vi "Front Lifter Control.vi"(11 "Go to Level?":i32) -> ()   [LabVIEW 2014]
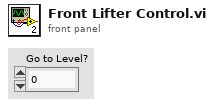
[diagram p1: front panel]
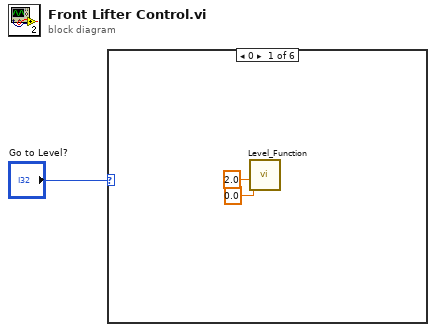
[diagram p0: block diagram]
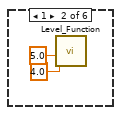
[diagram p2: hidden frame]
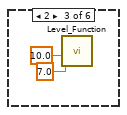
[diagram p3: hidden frame]
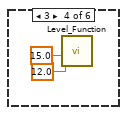
[diagram p4: hidden frame]
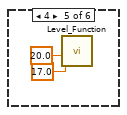
[diagram p5: hidden frame]
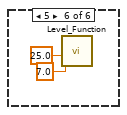
[diagram p6: hidden frame]
diagram:
  n1 = case shown="0" "Go to Level?" {
    frame 0 {
      n2 = call "Level_Function.vi"("lower Limit"=0.0, "upper limit"=2.0) -> ()  [unwired: 9 in, 1 out]
    }
    frame 1 {
      n3 = call "Level_Function.vi"("lower Limit"=4.0, "upper limit"=5.0) -> ()  [unwired: 9 in, 1 out]
    }
    frame 2 {
      n4 = call "Level_Function.vi"("lower Limit"=7.0, "upper limit"=10.0) -> ()  [unwired: 9 in, 1 out]
    }
    frame 3 {
      n5 = call "Level_Function.vi"("lower Limit"=12.0, "upper limit"=15.0) -> ()  [unwired: 9 in, 1 out]
    }
    frame 4 {
      n6 = call "Level_Function.vi"("lower Limit"=17.0, "upper limit"=20.0) -> ()  [unwired: 9 in, 1 out]
    }
    frame 5 {
      n7 = call "Level_Function.vi"("lower Limit"=7.0, "upper limit"=25.0) -> ()  [unwired: 9 in, 1 out]
    }
  }
